vi "omni lagtest.vi"() -> ()   [LabVIEW 2012, in "Omni2013.lvrbt"]
uses:
  Omni2013.lvrbt
  <vilib>/NXT/Hardware/Plugins/Tetrix DC Motor/TetrixDCMotorAddress.ctl
  <vilib>/NXT/Subs/MotorOutput.ctl
  <vilib>/NXT/Dual Mode Library/Display/drawNumber.vi
  <vilib>/NXT/Dual Mode Library/Display/drawNumber_float.vi
  <vilib>/NXT/NXTIO Xnodes/NXTIONodeSubVIs/TETRIX IO Move DC Motors.vi
  <vilib>/NXT/Dual Mode Library/Motors/MotorOn.vi
  <vilib>/NXT/Dual Mode Library/Motors/MotorBrake.vi
  <vilib>/NXT/Dual Mode Library/Motors/MotorReverse.vi
  <vilib>/NXT/Dual Mode Library/Display/drawText_Center.vi
  <vilib>/NXT/NXTIO Xnodes/AddressXNode/NXTIOAddress.xnode
  <vilib>/NXT/Subs/LVHSConnector.ctl
  <vilib>/NXT/NXTIO Xnodes/NXTIOXNode/NXTIO.xnode
  <vilib>/NXT/LegoClasses/BrickReference/BrickReference.lvclass
panel:
  in  "milSec#1":u32
  # "This VI was generated based on your configuration in the Remote Control Editor. You may modify the code as needed for your robot. To test this program for an FTC match, return to the Remote Control Editor, select the \"Run Program\" tab, and choose \"FTC Game\"."
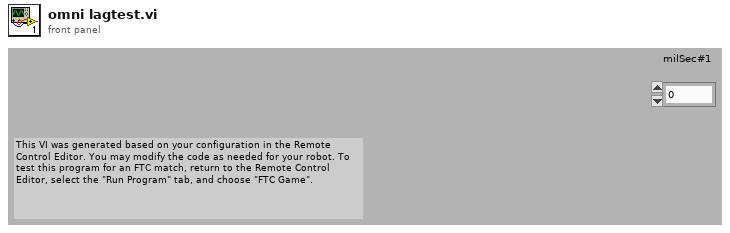
[diagram p1: front panel]
types:
  T1 = typedef "TetrixDCMotorAddress.ctl" = i16
  T2 = cluster{"TetrixDCMotor":T1, "TetrixDCMotor 2":T1}
  T3 = typedef "LVHSConnector.ctl" = refnum<class "BrickReference.lvclass">
  T4 = typedef "FTC ControllerState.ctl" = cluster{"Left X":i8, "Left Y":i8, "Right X":i8, "Right Y":i8, "Button Encoding 9-12":u8, "Button Encoding 1-8":u8, "POV":T5}
  T5 = typedef "FTC POVState.ctl" = i8
  T6 = typedef "FTC ButtonEventType.ctl" = enum16{"Pressed", "Released"}
  T7 = cluster{"Button ID":enum16{"None", "Button 1", "Button 2", "Button 3", "Button 4", "Button 5", "Button 6", "Button 7", "Button 8", "Button 9", "Button 10", "Button 11", "Button 12", "POV Up", "POV Up Right", "POV Right", "POV Down Right", "POV Down", "POV Down Left", "POV Left", "POV Up Left"}, "Event Type":T6}[]
  T8 = enum16{"None", "Button 1", "Button 2", "Button 3", "Button 4", "Button 5", "Button 6", "Button 7", "Button 8", "Button 9", "Button 10", "Button 11", "Button 12", "POV Up", "POV Up Right", "POV Right", "POV Down Right", "POV Down", "POV Down Left", "POV Left", "POV Up Left"}
  T9 = typedef "MotorOutput.ctl" = u8
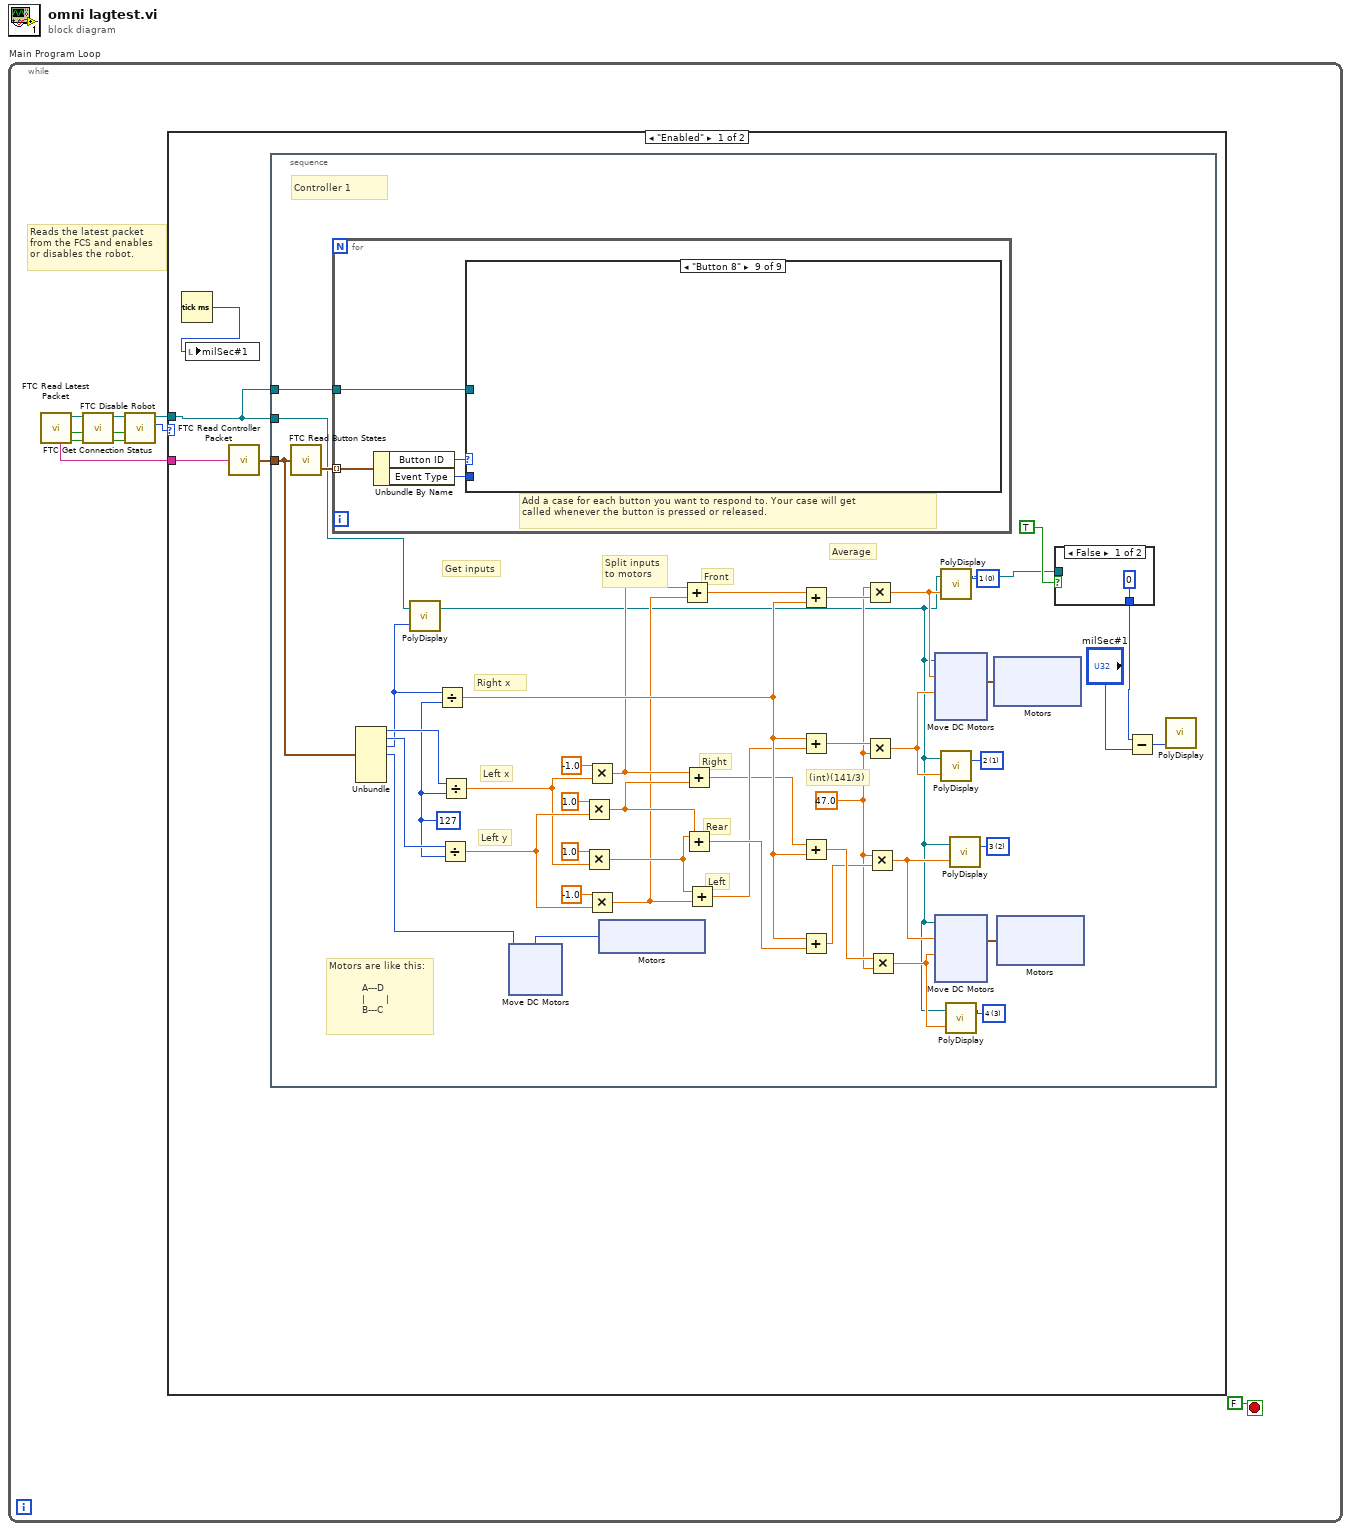
[diagram p0: block diagram]
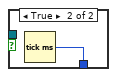
[diagram p2: hidden frame]
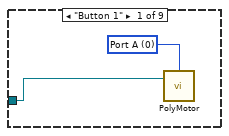
[diagram p3: hidden frame]
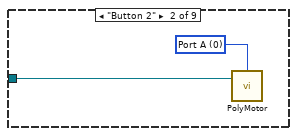
[diagram p4: hidden frame]
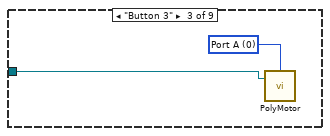
[diagram p5: hidden frame]
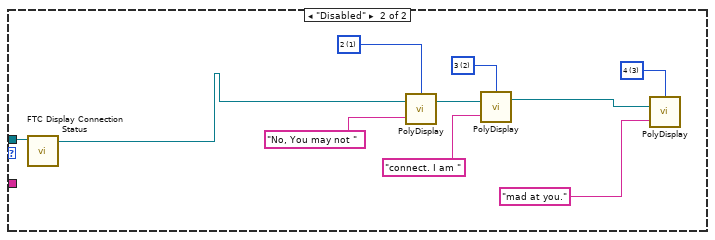
[diagram p11: hidden frame]
diagram:
  n1 = while "Main Program Loop" {
    stop <- FALSE stop-if-true
    # "Reads the latest packet\nfrom the FCS and enables\nor disables the robot."
    n2 = call <vilib>:"FTC Read Latest Packet.vi"() -> ("Packet Received?"=w8:bool, "Stopped?"=w5:bool, "NXT"=w7:T3, "Controller 1"=w9:string)  [unwired: 6 in, 2 out]
    n3 = call <vilib>:"FTC Get Connection Status.vi"("Packet Received?"=w8, "Stopped?"=w5, "NXT"=w7) -> ("Online?"=w2:bool, "Stopped?"=w3:bool, "NXT"=w4:T3)  [unwired: 5 in]
    n4 = call <vilib>:"FTC Disable Robot.vi"("Online?"=w2, "Stopped?"=w3, "NXT"=w4) -> ("Enabled?"=w6:enum16{"Disabled", "Enabled"}, "NXT"=w1:T3)  [unwired: 3 in]
    n5 = case "disableCase" shown="\"Enabled\"" w6 {
      tunnel: w9 -> [w14 _]
      tunnel: w1 -> [w12 w112]
      frame "Enabled" {
        n6 = Tick Count (ms)() -> (millisecond timer value=w11:u32)
        n7 = local write "milSec#1"(w11) -> ()
        n8 = call <vilib>:"FTC Read Controller Packet.vi"("Packet"=w14) -> ("Controller State"=w13:T4)  [unwired: 4 in]
        n9 = stacked-sequence "controller1Actions" {
          tunnel: w13 -> [w43]
          tunnel: w12 -> [w23]
          tunnel: w12 -> [w22]
          frame #0 {
            w33 = i8 127 ("y")
            w59 = i16 0 items=["1", "2", "3", "4", "5", "6", "7", "8"] ("Line")
            w58 = i16 3 items=["1", "2", "3", "4", "5", "6", "7", "8"] ("Line")
            w38 = i16 2 items=["1", "2", "3", "4", "5", "6", "7", "8"] ("Line")
            w57 = i16 1 items=["1", "2", "3", "4", "5", "6", "7", "8"] ("Line")
            w26 = 47.0 ("y")
            # "Average"
            # "Left"
            # "Rear"
            # "Right"
            # "Front"
            # "Motors are like this:\n\n           A---D\n           |       |\n           B---C"
            # "(int)(141/3)"
            # "Split inputs to motors"
            # "Get inputs"
            # "Left y"
            # "Right x"
            # "Left x"
            # "Controller 1"
            n10 = call <vilib>:"FTC Read Button States.vi"("Controller State"=w43) -> ("Button Events"=w60:T7)  [unwired: 2 in, 1 out]
            n11 = for "buttonAction" {
              tunnel: w60 -> [w94] mode=indexing
              tunnel: w23 -> [w93]
              # "Add a case for each button you want to respond to. Your case will get \ncalled whenever the button is pressed or released."
              n12 = Unbundle By Name(w94) -> ("Button ID"=w96:T8, "Event Type"=w95:T6)
              n13 = case "EventCase1" shown="\"Button 8\"" w96 {
                tunnel: w95 -> [_ _ _ _ _ _ _ _ _]
                tunnel: w93 -> [w97 w99 w101 _ _ _ _ _ _]
                frame "Button 1" {
                  w98 = T9 0 items=["Port A"=0, "Port B"=1, "Port C"=2, "Ports A & B"=4, "Ports A & C"=5, "Ports B & C"=6, "All Ports"=3] ("Output Port (All Ports)")
                  n14 = call-poly <vilib>:"PolyMotor.vi"("NXT"=w97, "Output Port (All Ports)"=w98) -> ()  [unwired: 2 in, 1 out]
                }
                frame "Button 2" {
                  w100 = T9 0 items=["Port A"=0, "Port B"=1, "Port C"=2, "Ports A & B"=4, "Ports A & C"=5, "Ports B & C"=6, "All Ports"=3] ("Output Port (All Ports)")
                  n15 = call-poly <vilib>:"PolyMotor.vi"("NXT"=w99, "Port (All Ports)"=w100) -> ()  [unwired: 2 in, 1 out]
                }
                frame "Button 3" {
                  w102 = T9 0 items=["Port A"=0, "Port B"=1, "Port C"=2, "Ports A & B"=4, "Ports A & C"=5, "Ports B & C"=6, "All Ports"=3] ("Output Port (All Ports)")
                  n16 = call-poly <vilib>:"PolyMotor.vi"("NXT"=w101, "Output Port (All Ports)"=w102) -> ()  [unwired: 2 in, 1 out]
                }
                frame "Button 4" {
                }
                frame Default {
                  # "No Action"
                }
                frame "Button 5" {
                }
                frame "Button 6" {
                }
                frame "Button 7" {
                }
                frame "Button 8" {
                }
              }
            }
            n17 = Unbundle(w43) -> ("Left X"=w34:i8, "Left Y"=w35:i8, "Right X"=w21:i8, "Right Y"=w24:i8)  [unwired: 3 out]
            n18 = call-poly <vilib>:"PolyDisplay.vi"("number"=w21, "NXT"=w22) -> ("NXT"=w19:T3)  [unwired: 2 in]
            n19 = Divide(x=w21, y=w33) -> (x/y=w55:dbl)
            n20 = Divide(x=w35, y=w33) -> (x/y=w49:dbl)
            n21 = Divide(x=w34, y=w33) -> (x/y=w46:dbl)
            n22 = Multiply(x=1.0, y=w49) -> (x*y=w32:dbl)
            n23 = Multiply(x=1.0, y=w46) -> (x*y=w50:dbl)
            n24 = Multiply(x=-1.0, y=w46) -> (x*y=w51:dbl)
            n25 = Multiply(x=-1.0, y=w49) -> (x*y=w31:dbl)
            n26 = xnode "Motors"() -> ("Motor"=w25:T1)
            n27 = xnode "Move DC Motors"("Power/Speed 1"=w24, "Motors"=w25) -> ()  [unwired: 1 in, 1 out]
            n28 = Add(x=w51, y=w31) -> (x+y=w54:dbl)
            n29 = Add(x=w51, y=w32) -> (x+y=w52:dbl)
            n30 = Add(x=w50, y=w32) -> (x+y=w56:dbl)
            n31 = Add(x=w50, y=w31) -> (x+y=w53:dbl)
            n32 = Add(x=w54, y=w55) -> (x+y=w28:dbl)
            n33 = Add(x=w55, y=w53) -> (x+y=w29:dbl)
            n34 = Add(x=w52, y=w55) -> (x+y=w30:dbl)
            n35 = Add(x=w55, y=w56) -> (x+y=w27:dbl)
            n36 = Multiply(x=w26, y=w28) -> (x*y=w41:dbl)
            n37 = Multiply(x=w29, y=w26) -> (x*y=w40:dbl)
            n38 = Multiply(x=w26, y=w27) -> (x*y=w36:dbl)
            n39 = Multiply(x=w30, y=w26) -> (x*y=w37:dbl)
            n40 = call-poly <vilib>:"PolyDisplay.vi"("number"=w41, "NXT"=w19, "Line"=w59) -> ("NXT"=w18:T3)  [unwired: 1 in]
            n41 = call-poly <vilib>:"PolyDisplay.vi"("number"=w40, "NXT"=w19, "Line"=w57) -> ()  [unwired: 1 in, 1 out]
            n42 = call-poly <vilib>:"PolyDisplay.vi"("number"=w37, "NXT"=w19, "Line"=w58) -> ()  [unwired: 1 in, 1 out]
            n43 = call-poly <vilib>:"PolyDisplay.vi"("number"=w36, "NXT"=w19, "Line"=w38) -> ()  [unwired: 1 in, 1 out]
            n44 = xnode "Motors"() -> ("Motor"=w42:cluster{"TetrixDCMotor":T1, "TetrixDCMotor":T1})
            n45 = xnode "Move DC Motors"("Power/Speed 2"=w40, "Power/Speed 1"=w41, "Motors"=w42, "NXT"=w19) -> ()  [unwired: 1 out]
            n46 = xnode "Motors"() -> ("Motor"=w39:cluster{"TetrixDCMotor":T1, "TetrixDCMotor":T1})
            n47 = xnode "Move DC Motors"("Power/Speed 2"=w37, "Power/Speed 1"=w36, "Motors"=w39, "NXT"=w19) -> ()  [unwired: 1 out]
            n48 = case shown="False" TRUE {
              tunnel: w18 -> [_ _]
              tunnel: [u32 0 ("millisecond timer value") w62] -> w17
              frame False {
              }
              frame True {
                n49 = Tick Count (ms)() -> (millisecond timer value=w62:u32)
              }
            }
            n50 = Subtract(x=w17, y="milSec#1") -> (x-y=w15:u32)
            n51 = call-poly <vilib>:"PolyDisplay.vi"("number"=w15) -> ()  [unwired: 3 in, 1 out]
          }
        }
      }
      frame "Disabled" {
        w105 = i16 3 items=["1", "2", "3", "4", "5", "6", "7", "8"] ("Line")
        w111 = i16 2 items=["1", "2", "3", "4", "5", "6", "7", "8"] ("Line")
        w107 = i16 1 items=["1", "2", "3", "4", "5", "6", "7", "8"] ("Line")
        n52 = call <vilib>:"FTC Display Connection Status.vi"("NXT"=w112) -> ("NXT"=w106:T3)  [unwired: 10 in]
        n53 = call-poly <vilib>:"PolyDisplay.vi"("Text"="No, You may not ", "NXT"=w106, "Line"=w107) -> ("NXT"=w109:T3)  [unwired: 1 in]
        n54 = call-poly <vilib>:"PolyDisplay.vi"("Text"="connect. I am ", "NXT"=w109, "Line"=w111) -> ("NXT"=w104:T3)  [unwired: 1 in]
        n55 = call-poly <vilib>:"PolyDisplay.vi"("Text"="mad at you.", "NXT"=w104, "Line"=w105) -> ()  [unwired: 1 in, 1 out]
      }
    }
  }
